vi "ProcessResults.vi"(10 "Response Array":T1[](array[typedef])) -> (2 "True Response":T1[](array[typedef]))   [LabVIEW 2020, in "Controller.lvlib"]
uses:
  Controller.lvlib
  Public Controls/IP Address Response Type Def.ctl
  UI/UI.lvlib
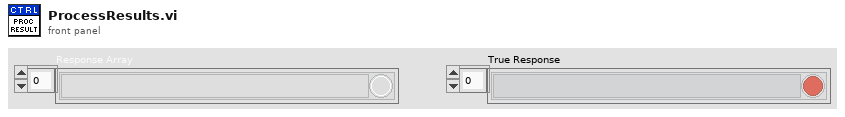
[diagram p1: front panel]
types:
  T1 = typedef "UI.lvlib/IP Address Response Type Def.ctl" = cluster{"Response":string, "Boolean":bool}
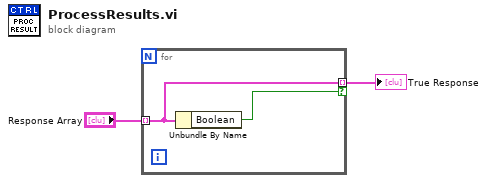
[diagram p0: block diagram]
diagram:
  n1 = for {
    tunnel: "Response Array" -> [w4] mode=indexing
    tunnel: [w4] -> w1 mode=indexing if=w3
    n2 = Unbundle By Name(w4) -> ("Boolean"=w3:bool)
  }
  "True Response" <- w1
